vi "HEWH RLT Get Current.vi"(8 "Error In":errorcluster, 9 "DAQ for A":bool, 10 "A Data Array":string[][](array[string])) -> (0 "Error Out":errorcluster, 3 "Current":dbl)   [LabVIEW 2016]
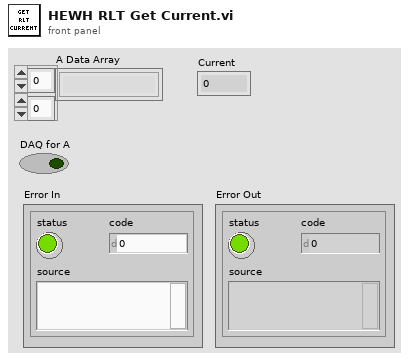
[diagram p1: front panel]
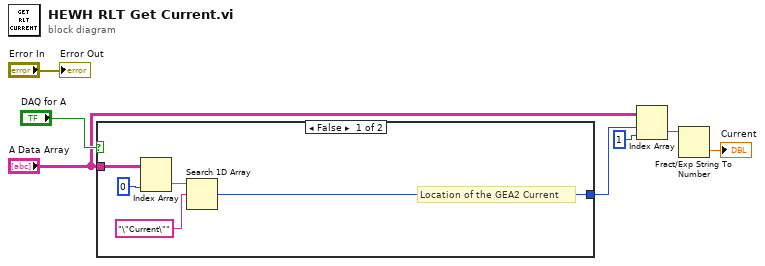
[diagram p0: block diagram]
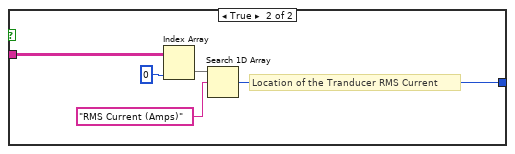
[diagram p2: hidden frame]
diagram:
  n1 = case shown="False" "DAQ for A" {
    tunnel: [w8 w13] -> w3
    tunnel: "A Data Array" -> [w9 w14]
    frame False {
      # "Location of the GEA2 Current"
      n2 = Index Array(array=w9, index (col)=0 ("disabled index (col)")) -> (element=w11:string[])  [unwired: 1 in]
      n3 = Search 1D Array(1D array=w11, element="\"Current\"") -> (index of element=w8:i32)  [unwired: 1 in]
    }
    frame True {
      # "Location of the Tranducer RMS Current"
      n4 = Index Array(array=w14, index (col)=0 ("disabled index (col)")) -> (element=w16:string[])  [unwired: 1 in]
      n5 = Search 1D Array(1D array=w16, element="RMS Current (Amps)") -> (index of element=w13:i32)  [unwired: 1 in]
    }
  }
  n6 = Index Array(array="A Data Array", index (row)=w3, index (col)=1 ("disabled index (col)")) -> (element=w2:string)
  n7 = Fract/Exp String To Number(string=w2) -> (number=→"Current":dbl)  [unwired: 3 in, 1 out]
  "Error Out" <- "Error In"
